vi "real-time recording.vi"() -> ()   [LabVIEW 2012]
doc: "This VI will initialize the FPGA VI and read a user-defined number of samples from a DMA FIFO. When the data acquisition is complete this VI will read status information from the FPGA VI.\n\nFollow these instructions to run the VI.\n\n1. Select your RIO device from the dropdown.\n2. Set the sample period, number of samples to acquire per channel, and DMA block read size. \n\nNote: the block read size should be set to balance load on the host processor and the update rate of the user interface. A small block read size will update the user interface more often but will result in a higher load on the host processor."
uses:
  <vilib>/userdefined/High Color/nirio_resource_hc.ctl
  <vilib>/Analysis/3filter.llb/Butterworth Filter (DBL).vi
  <vilib>/FPGAPlugInAG/sbRIO-9612/niLvFpga_Open_sbRIO-9612.vi
  <vilib>/rvi/interface/common/dynamic/niFpgaDynamicAddResources.vi
  <vilib>/Utility/error.llb/Error Cluster From Error Code.vi
  <vilib>/FPGAPlugInAG/Dynamic/niLvFpga_Run_Dynamic.vi
  <vilib>/rvi/errors/niLvFpgaAdjustHostInterfaceError.vi
  <vilib>/RVI Host/nirviSupport.llb/nirviErrorClusterFromErrorCode.vi
  <vilib>/FPGAPlugInAG/Dynamic/niLvFpga_Close_Dynamic.vi
  <vilib>/rvi/interface/nirviOpenFPGA/nirviOpenFPGA.xnode
  FPGA Bitfiles/bbauvFPGA_FPGATarget2_NI9223User-Contr_AXBjtBmtN8Y.lvbitx
  NI 9223 User-Controlled IO Sampling (FPGA).vi
  <vilib>/rvi/interface/nirviMethod/nirviMethod.xnode
  <vilib>/rvi/interface/nirviReadWriteControl/nirviReadWriteControl.xnode
  <vilib>/rvi/interface/nirviCloseFPGA/nirviCloseFPGA.xnode
  <vilib>/rvi/errors/niLvFpgaMergeErrorWithErrorCode.vi
  <vilib>/rvi/interface/Simulation/niFpgaSimulationCallBeginRW.vi
  <vilib>/FPGAPlugInAG/Dynamic/niLvFpga_ReadFifo_Dynamic.vi
  <vilib>/rvi/interface/nirviMethod/StockFPGA_InlinedMethodWaitForSingleIRQ.vi
  <vilib>/FPGAPlugInAG/Dynamic/niLvFpga_WaitOnIrq_Dynamic.vi
  <vilib>/FPGAPlugInAG/Dynamic/niLvFpga_AcknowledgeIrq_Dynamic.vi
  NiFpgaLv.dll
  <vilib>/FPGAPlugInAG/Dynamic/niLvFpga_ConfigureFifo_Dynamic.vi
  <vilib>/FPGAPlugInAG/Dynamic/niLvFpga_StartFifo_Dynamic.vi
  <vilib>/Analysis/NI_AALBase.lvlib
  <vilib>/Analysis/NI_AALPro.lvlib
panel:
  in  "fake dt2":dbl
  in  "Record?":bool
  in  "Filename":path=path "D/Recorded/US Test/Record 1/test 1.tdms"
  in  "threshold ratio":dbl=3.0
  out "Sidemove":dbl
  out "Forward":dbl
  out "Threshold 3":dbl
  out "Threshold 2":dbl
  out "Threshold 1":dbl
  out "noise index":dbl[](array[numeric])
  out "Threshold 0":dbl
  out "Amplitude Spectrum":waveform(dbl)(graph)
  out "bad signal?":bool
  in  "Min Starting Index":i32=7000
  in  "Portion Duration":i32=1000
  out "amplitude 3":dbl
  out "amplitude 2":dbl
  out "amplitude 1":dbl
  out "amplitude 0":dbl
  in  "noise min":dbl=0.001
  out "Index 3":dbl
  out "Index 2":dbl
  out "Index 1":dbl
  out "Index 0":dbl
  out "current time":timestamp
  in  "Debug":bool=TRUE
  in  "Send to ROS":bool
  out "ROS  Error":bool
  out "dt1":dbl
  out "dt2":dbl
  out "dt3":dbl
  out "pitch":dbl
  out "yaw":dbl
  out "z":dbl
  out "y":dbl
  out "x":dbl
  in  "Mode":T1(ring)=enum."Use Far Field"
  in  "Altitude":dbl=2.0
  in  "Display Filtered Signal":bool=TRUE
  out "Ratio at Index (%)":dbl
  out "Selected Index":i32
  in  "Threshold":dbl=0.1
  in  "low cutoff freq: fl":dbl=20000.0
  in  "high cutoff freq: fh":dbl=30000.0
  out "Yaw Chart":dbl(graph)
  out "Ch0 Signal":dbl[](graph)
  out "#Elements Acquired":u32(graph)
  out "Extracted signal":dbl[][](graph)
  in  "Sampling Duration (us)":u32=2005000
  in  "RIO Device":T2="rio://192.168.0.150/RIO0"
  out "Timed Out":bool
  out "Sample Gated":bool
  out "Overwrite":bool
  in  "Acquisition Stop":bool
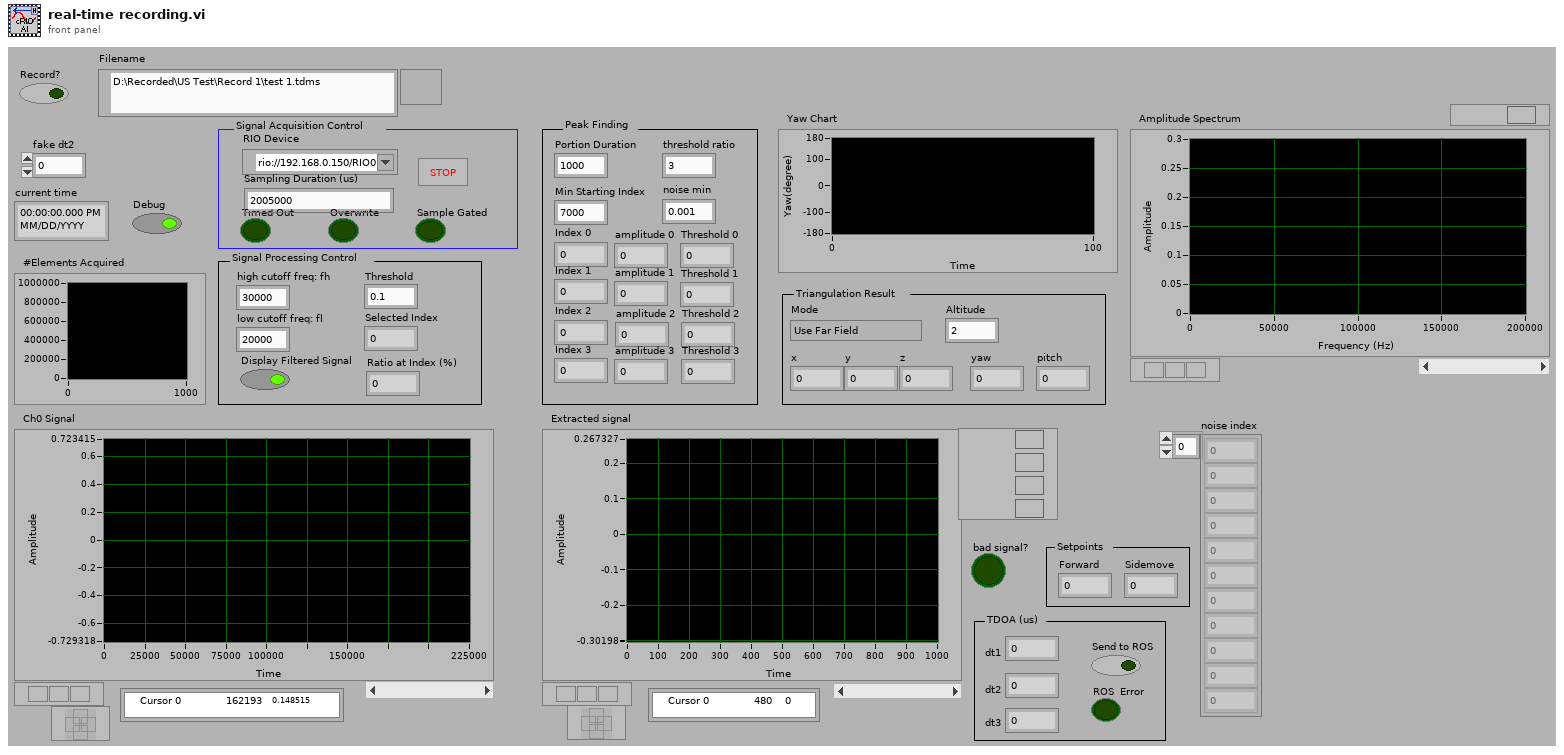
[diagram p1: front panel]
types:
  T1 = enum16{"Use Near Field", "Use Far Field", "Far Field with 3 hydrophones"}
  T2 = typedef "nirio_resource_hc.ctl" = tag
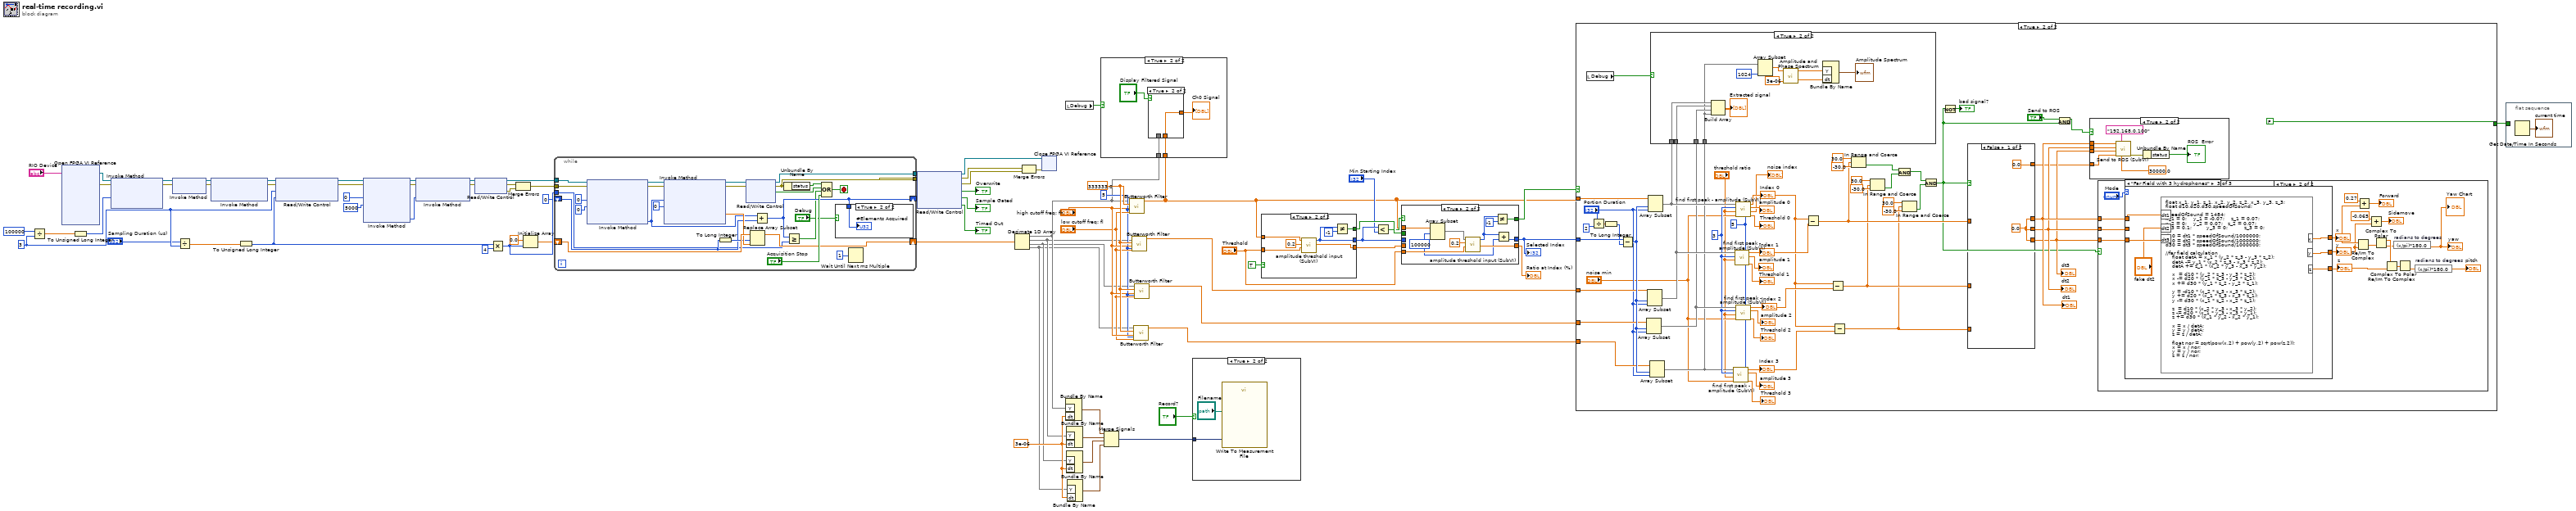
[diagram p0: block diagram]
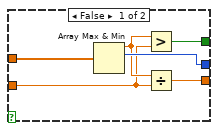
[diagram p6: hidden frame]
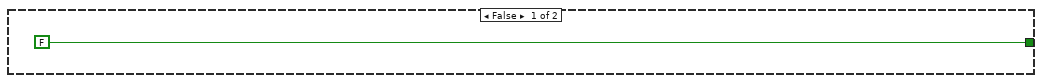
[diagram p7: hidden frame]
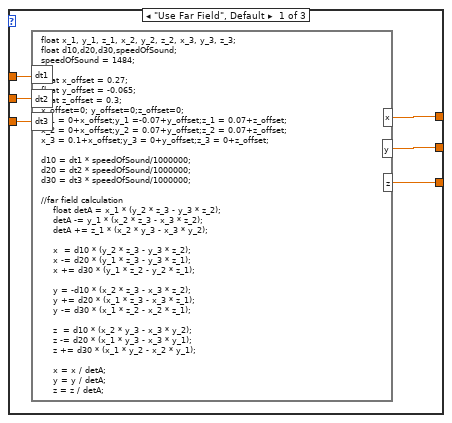
[diagram p9: hidden frame]
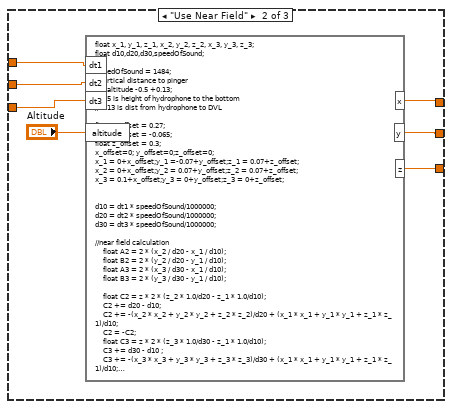
[diagram p10: hidden frame]
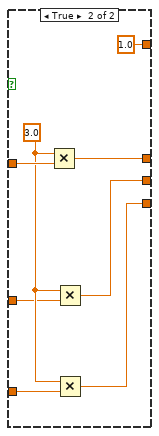
[diagram p12: hidden frame]
diagram:
  w8 = 3e-06
  w16 = 5
  w22 = 333333.0
  w36 = u32 3
  n1 = Divide(x=u32 100000, y=w36) -> (x/y=w69:dbl)
  n2 = xnode "Open FPGA VI Reference"("resource name"="RIO Device") -> ("FPGA VI Reference Out"=w72:refnum<k20>, "error out"=w71:errorcluster)  [unwired: 1 in]
  n3 = To Unsigned Long Integer(number=w69) -> (unsigned 32bit integer=w70:u32)
  n4 = xnode "Invoke Method"("FPGA VI Reference In"=w72, "error in"=w71, "Requested Depth"=w70) -> ("FPGA VI Reference Out"=w74:refnum<k20>, "error out"=w73:errorcluster)  [unwired: 1 out]
  n5 = xnode "Invoke Method"("FPGA VI Reference In"=w74, "error in"=w73) -> ("FPGA VI Reference Out"=w63:refnum<k20>, "error out"=w62:errorcluster)
  n6 = Divide(x="Sampling Duration (us)", y=w36) -> (x/y=w34:dbl)
  n7 = xnode "Invoke Method"("FPGA VI Reference In"=w63, "error in"=w62) -> ("FPGA VI Reference Out"=w39:refnum<k20>, "error out"=w38:errorcluster)  [unwired: 1 in]
  n8 = To Unsigned Long Integer(number=w34) -> (unsigned 32bit integer=w32:u32)
  n9 = xnode "Read/Write Control"("FPGA VI Reference In"=w39, "error in"=w38, "Sample Period (uSec)"=w36, "Number of Samples"=w32) -> ("FPGA VI Reference Out"=w53:refnum<k20>, "error out"=w52:errorcluster)
  n10 = xnode "Invoke Method"("FPGA VI Reference In"=w53, "error in"=w52, "IRQ Number(s)"=0, "Timeout (ms)"=5000) -> ("FPGA VI Reference Out"=w50:refnum<k20>, "error out"=w51:errorcluster, "IRQ(s) Asserted"=w47:i32)  [unwired: 1 out]
  n11 = xnode "Invoke Method"("FPGA VI Reference In"=w50, "error in"=w51, "IRQ Number(s)"=w47) -> ("FPGA VI Reference Out"=w49:refnum<k20>, "error out"=w48:errorcluster)
  n12 = xnode "Read/Write Control"("FPGA VI Reference In"=w49, "error in"=w48) -> ("FPGA VI Reference Out"=w41:refnum<k20>, "error out"=w55:errorcluster, "Error Out"=w54:errorcluster)
  n13 = Multiply(x=w32, y=u32 4) -> (x*y=w66:u32)
  n14 = Merge Errors(w55, w54) -> (w40:errorcluster)
  n15 = Initialize Array(sgl 0.0, w66) -> (w42:sgl[])
  n16 = while {
    tunnel: w41 -> [w88]
    tunnel: w40 -> [w87]
    tunnel: [w96] -> w61
    tunnel: [w95] -> w60
    shift-right: [w78] -> _
    shift-left: u32 0 -> [w89]
    tunnel: w66 -> [w81]
    shift-right: [w91] -> w33
    shift-left: w42 -> [w97]
    stop <- w98 stop-if-true
    n17 = xnode "Invoke Method"("FPGA VI Reference In"=w88, "error in"=w87, "Number of Elements"=u32 0, "Timeout (ms)"=0) -> ("FPGA VI Reference Out"=w86:refnum<k20>, "error out"=w85:errorcluster, "Elements Remaining"=w79:u32)  [unwired: 1 out]
    n18 = xnode "Invoke Method"("FPGA VI Reference In"=w86, "error in"=w85, "Number of Elements"=w79, "Timeout (ms)"=0) -> ("FPGA VI Reference Out"=w101:refnum<k20>, "error out"=w100:errorcluster, "Data"=w92:sgl[])  [unwired: 1 out]
    n19 = To Long Integer(number=w89) -> (32bit integer=w90:i32)
    n20 = xnode "Read/Write Control"("FPGA VI Reference In"=w101, "error in"=w100) -> ("FPGA VI Reference Out"=w96:refnum<k20>, "error out"=w95:errorcluster, "Error"=w80:bool)  [unwired: 1 out]
    n21 = Replace Array Subset(array=w97, new element=w92, index=w90) -> (w91:sgl[])
    n22 = Add(x=w79, y=w89) -> (x+y=w78:u32)
    n23 = Unbundle By Name(w95) -> ("status"=w82:bool)
    n24 = Greater Or Equal?(x=w78, y=w81) -> (x >= y?=w77:bool)
    n25 = Compound Arithmetic op=OR(w82, w80, w77, "Acquisition Stop") -> (w98:bool)
    n26 = case shown="True" "Debug" {
      tunnel: w78 -> [_ w102]
      frame False {
      }
      frame True {
        "#Elements Acquired" <- w102
      }
    }
    n27 = Wait Until Next ms Multiple(millisecond multiple=u32 1) -> ()  [unwired: 1 out]
  }
  n28 = xnode "Read/Write Control"("FPGA VI Reference In"=w61, "error in"=w60) -> ("FPGA VI Reference Out"=w65:refnum<k20>, "error out"=w56:errorcluster, "Error Out"=w57:errorcluster, "Overwrite"=→"Overwrite":bool, "Sample Gated"=→"Sample Gated":bool, "Timed Out"=→"Timed Out":bool)
  n29 = Decimate 1D Array(w33) -> (w4:sgl[], w3:sgl[], w2:sgl[], w1:sgl[])
  n30 = Merge Errors(w56, w57) -> (w64:errorcluster)
  n31 = xnode "Close FPGA VI Reference"("FPGA VI Reference In"=w65, "error in"=w64) -> ()  [unwired: 1 out]
  n32 = local read "Debug"() -> (w14:bool)
  n33 = Bundle By Name("Y"=w4, "dt"=w8) -> (w11:waveform(sgl))  [unwired: 1 in]
  n34 = Bundle By Name("Y"=w3, "dt"=w8) -> (w10:waveform(sgl))  [unwired: 1 in]
  n35 = Bundle By Name("Y"=w2, "dt"=w8) -> (w9:waveform(sgl))  [unwired: 1 in]
  n36 = Bundle By Name("Y"=w1, "dt"=w8) -> (w7:waveform(sgl))  [unwired: 1 in]
  n37 = Merge Signals(w11, w10, w9, w7) -> (w6:dynamicdata)
  n38 = call-poly <vilib>:"Butterworth Filter.vi"("order"=w16, "low cutoff freq: fl"="low cutoff freq: fl", "high cutoff freq: fh"="high cutoff freq: fh", "sampling freq: fs"=w22, "X"=w4) -> ("Filtered X"=w12:dbl[])  [unwired: 3 in, 1 out]
  n39 = case shown="True" w14 {
    tunnel: w12 -> [_ w104]
    tunnel: w4 -> [_ w103]
    frame False {
    }
    frame True {
      n40 = case shown="True" "Display Filtered Signal" {
        tunnel: w103 -> [w107 _]
        tunnel: [w107 w108] -> w105
        tunnel: w104 -> [_ w108]
        frame False {
        }
        frame True {
        }
      }
      "Ch0 Signal" <- w105
    }
  }
  n41 = call-poly <vilib>:"Butterworth Filter.vi"("order"=w16, "low cutoff freq: fl"="low cutoff freq: fl", "high cutoff freq: fh"="high cutoff freq: fh", "sampling freq: fs"=w22, "X"=w3) -> ("Filtered X"=w19:dbl[])  [unwired: 3 in, 1 out]
  n42 = call-poly <vilib>:"Butterworth Filter.vi"("order"=w16, "low cutoff freq: fl"="low cutoff freq: fl", "high cutoff freq: fh"="high cutoff freq: fh", "sampling freq: fs"=w22, "X"=w1) -> ("Filtered X"=w17:dbl[])  [unwired: 3 in, 1 out]
  n43 = call-poly <vilib>:"Butterworth Filter.vi"("order"=w16, "low cutoff freq: fl"="low cutoff freq: fl", "high cutoff freq: fh"="high cutoff freq: fh", "sampling freq: fs"=w22, "X"=w2) -> ("Filtered X"=w18:dbl[])  [unwired: 3 in, 1 out]
  n44 = case shown="True" "Record?" {
    tunnel: w6 -> [_ w110]
    frame False {
    }
    frame True {
      n45 = call "Write To Measurement File"("Signals"=w110, "Filename"="Filename") -> ()  [unwired: 15 in, 3 out]
    }
  }
  n46 = case shown="True" TRUE {
    tunnel: w12 -> [w116 w123]
    tunnel: [w113 w120] -> w28
    tunnel: [w114 w119] -> w25
    tunnel: [w115 w118] -> w30
    tunnel: "Threshold" -> [w111 w117]
    frame False {
      n47 = Array Max & Min(array=w116) -> (max value=w112:dbl, max index (indices)=w114:i32)  [unwired: 2 out]
      n48 = Greater?(x=w112, y=w111) -> (0:w115:bool)
      n49 = Divide(x=w112, y=w111) -> (x/y=w113:dbl)
    }
    frame True {
      n50 = call "amplitude threshold input (SubVI).vi"("threshold"=w117, "%max amplitude"=0.2, "Array"=w123) -> ("actual ratio (%)"=w120:dbl, "Index"=w119:i32)  [unwired: 7 in]
      n51 = Not Equal?(x=w119, y=-1) -> (x != y?=w118:bool)
    }
  }
  n52 = Less?(x=w25, y="Min Starting Index") -> (x < y?=w29:bool)
  n53 = case shown="True" w29 {
    tunnel: w30 -> [w126 _]
    tunnel: w28 -> [w124 _]
    tunnel: w12 -> [_ w136]
    tunnel: "Threshold" -> [_ w132]
    tunnel: [w126 w131] -> w23
    tunnel: [w125 w129] -> w24
    tunnel: [w124 w130] -> w26
    tunnel: w25 -> [w125 _]
    frame False {
    }
    frame True {
      w127 = 100000
      n54 = Array Subset(array=w136, index=w127) -> (w133:dbl[])  [unwired: 1 in]
      n55 = call "amplitude threshold input (SubVI).vi"("threshold"=w132, "%max amplitude"=0.2, "Array"=w133) -> ("actual ratio (%)"=w130:dbl, "Index"=w128:i32)  [unwired: 7 in]
      n56 = Not Equal?(x=w128, y=-1) -> (x != y?=w131:bool)
      n57 = Add(x=w128, y=w127) -> (x+y=w129:i32)
    }
  }
  "Ratio at Index (%)" <- w26
  "Selected Index" <- w24
  n58 = case shown="True" w23 {
    tunnel: w19 -> [_ w190]
    tunnel: w18 -> [_ w189]
    tunnel: w17 -> [_ w188]
    tunnel: w12 -> [_ w187]
    tunnel: w24 -> [_ w186]
    tunnel: [FALSE FALSE] -> w13
    frame False {
    }
    frame True {
      w138 = 5
      w151 = 3
      n59 = local read "Debug"() -> (w181:bool)
      n60 = Divide(x="Portion Duration", y=2) -> (x/y=w183:dbl)
      n61 = To Long Integer(number=w183) -> (32bit integer=w182:i32)
      n62 = Subtract(x=w186, y=w182) -> (x-y=w191:i32)
      n63 = Array Subset(array=w189, index=w191, length="Portion Duration") -> (w152:dbl[])
      n64 = Array Subset(array=w190, index=w191, length="Portion Duration") -> (w156:dbl[])
      n65 = Array Subset(array=w187, index=w191, length="Portion Duration") -> (w158:dbl[])
      n66 = Array Subset(array=w188, index=w191, length="Portion Duration") -> (w150:dbl[])
      n67 = case shown="True" w181 {
        tunnel: w156 -> [_ w257]
        tunnel: w152 -> [_ w256]
        tunnel: w150 -> [_ w247]
        tunnel: w158 -> [_ w255]
        frame False {
        }
        frame True {
          n68 = Build Array(w255, w257, w256, w247) -> (→"Extracted signal":dbl[][])
          n69 = Array Subset(array=w247, length=1024) -> (w251:dbl[])  [unwired: 1 in]
          n70 = call <vilib>:"Amplitude and Phase Spectrum.vi"("dt"=3e-06, "Signal (V)"=w251) -> ("df"=w248:dbl, "Amp Spectrum Mag (Vrms)"=w249:dbl[])  [unwired: 1 in, 1 out]
          n71 = Bundle By Name("Y"=w249, "dt"=w248) -> (→"Amplitude Spectrum":waveform(dbl))  [unwired: 1 in]
        }
      }
      n72 = call "find first peak - amplitude (SubVI).vi"("Noise length"=w138, "Noise min"="noise min", "threshold ratio"="threshold ratio", "width"=w151, "Array"=w150) -> ("Peak threshold"=→"Threshold 3":dbl, "peak amplitude"=→"amplitude 3":dbl, "Index"=w149:dbl)  [unwired: 2 in, 2 out]
      "Index 3" <- w149
      n73 = call "find first peak - amplitude (SubVI).vi"("Noise length"=w138, "threshold ratio"="threshold ratio", "width"=w151, "Array"=w156) -> ("Peak threshold"=→"Threshold 1":dbl, "peak amplitude"=→"amplitude 1":dbl, "Index"=w155:dbl)  [unwired: 3 in, 2 out]
      "Index 1" <- w155
      n74 = call "find first peak - amplitude (SubVI).vi"("Noise length"=w138, "Noise min"="noise min", "threshold ratio"="threshold ratio", "width"=w151, "Array"=w158) -> ("Peak threshold"=→"Threshold 0":dbl, "noise index"=→"noise index":dbl[], "peak amplitude"=→"amplitude 0":dbl, "Index"=w145:dbl)  [unwired: 2 in, 1 out]
      "Index 0" <- w145
      n75 = call "find first peak - amplitude (SubVI).vi"("Noise length"=w138, "Noise min"="noise min", "threshold ratio"="threshold ratio", "width"=w151, "Array"=w152) -> ("Peak threshold"=→"Threshold 2":dbl, "peak amplitude"=→"amplitude 2":dbl, "Index"=w153:dbl)  [unwired: 2 in, 2 out]
      "Index 2" <- w153
      n76 = Subtract(x=w145, y=w155) -> (x-y=w177:dbl)
      n77 = Subtract(x=w145, y=w153) -> (x-y=w174:dbl)
      n78 = Subtract(x=w145, y=w149) -> (x-y=w171:dbl)
      n79 = In Range and Coerce(upper limit=30.0, x=w177, lower limit=-30.0) -> (In Range?=w170:bool)  [unwired: 1 out]
      n80 = In Range and Coerce(upper limit=30.0, x=w174, lower limit=-30.0) -> (In Range?=w169:bool)  [unwired: 1 out]
      n81 = And(x=w170, y=w169) -> (x .and. y?=w168:bool)
      n82 = In Range and Coerce(upper limit=30.0, x=w171, lower limit=-30.0) -> (In Range?=w167:bool)  [unwired: 1 out]
      n83 = And(x=w168, y=w167) -> (x .and. y?=w159:bool)
      n84 = Not(x=w159) -> (.not. x?=→"bad signal?":bool)
      n85 = case shown="False" w159 {
        tunnel: w177 -> [_ w246]
        tunnel: w174 -> [_ w244]
        tunnel: w171 -> [_ w243]
        tunnel: [w237 w242] -> w164
        tunnel: [w237 w241] -> w163
        tunnel: [w237 w240] -> w162
        tunnel: [0.0 1.0] -> w161
        frame False {
          w237 = 0.0
        }
        frame True {
          w245 = 3.0
          n86 = Multiply(x=w245, y=w246) -> (x*y=w242:dbl)
          n87 = Multiply(x=w245, y=w244) -> (x*y=w241:dbl)
          n88 = Multiply(x=w245, y=w243) -> (x*y=w240:dbl)
        }
      }
      "dt1" <- w164
      "dt2" <- w163
      "dt3" <- w162
      n89 = And(x="Send to ROS", y=w159) -> (x .and. y?=w160:bool)
      n90 = case shown="True" w160 {
        tunnel: w164 -> [_ w232]
        tunnel: w163 -> [_ w231]
        tunnel: w162 -> [_ w230]
        tunnel: w161 -> [_ w229]
        frame False {
        }
        frame True {
          n91 = call "Send to ROS (SubVI).vi"("frequency"=30000.0, "ROS IP"="192.168.0.100", "Good signal?"=w229, "dt 3"=w230, "dt2"=w231, "dt 1"=w232) -> ("error out"=w235:errorcluster)  [unwired: 5 in]
          n92 = Unbundle By Name(w235) -> ("status"=→"ROS  Error":bool)
        }
      }
      n93 = case shown="True" w159 {
        tunnel: w164 -> [_ w200]
        tunnel: w163 -> [_ w199]
        tunnel: w162 -> [_ w198]
        frame False {
        }
        frame True {
          n94 = case shown="\"Far Field with 3 hydrophones\"" "Mode" {
            tunnel: [w215 w222 w228] -> w197
            tunnel: [w214 w221 w227] -> w194
            tunnel: [w213 w220 w226] -> w204
            tunnel: w200 -> [w212 w218 w225]
            tunnel: w199 -> [w211 w217 _]
            tunnel: w198 -> [w210 w216 w224]
            frame "Use Far Field", Default {
              n95 = formula code="float x_1, y_1, z_1, x_2, y_2, z_2, x_3, y_3, z_3;\nfloat d10,d20,d30,speedOfSound;\nspeedOfSound = 1484;\n\nfloat x_offset = 0.27;\nfloat y_offset = -0.065;\nfloat z_offset = 0.3;\nx_offset=0; y_offset=0;z_offset=0;\nx_1 = 0+x_offset;y_1 =-0.07+y_offset;z_1 = 0.07+z_offset;\nx_2 = 0+x_offset;y_2 = 0.07+y_offset;z_2 = 0.07+z_offset;\nx_3 = 0.1+x_offset;y_3 = 0+y_offset;z_3 = 0+z_offset;\n\nd10 = dt1 * speedOfSound/1000000;\nd20 = dt2 * speedOfSound/1000000;\nd30 = dt3 * speedOfSound/1000000;\n\n//far field calculation\n    float detA = x_1 * (y_2 * z_3 - y_3 * z_2);\n    detA -= y_1 * (x_2 * z_3 - x_3 * z_2);\n    detA += z_1 * (x_2 * y_3 - x_3 * y_2);\n\n    x  = d10 * (y_2 * z_3 - y_3 * z_2);\n    x -= d20 * (y_1 * z_3 - y_3 * z_1);\n    x += d30 * (y_1 * z_2 - y_2 * z_1);\n\n    y = -d10 * (x_2 * z_3 - x_3 * z_2);\n    y += d20 * (x_1 * z_3 - x_3 * z_1);\n    y -= d30 * (x_1 * z_2 - x_2 * z_1);\n\n    z  = d10 * (x_2 * y_3 - x_3 * y_2);\n    z -= d20 * (x_1 * y_3 - x_3 * y_1);\n    z += d30 * (x_1 * y_2 - x_2 * y_1);\n\n    x = x / detA;\n    y = y / detA;\n    z = z / detA;\n\n    float nor = sqrt(pow(x,2) + pow(y,2) + pow(z,2));\n    x = x / nor;\n    y = y / nor;\n    z = z / nor;"("dt1"=w212, "dt2"=w211, "dt3"=w210) -> ("x"=w215:dbl, "y"=w214:dbl, "z"=w213:dbl)
            }
            frame "Use Near Field" {
              n96 = formula code="float x_1, y_1, z_1, x_2, y_2, z_2, x_3, y_3, z_3;\nfloat d10,d20,d30,speedOfSound;\n\nspeedOfSound = 1484;\n//vertical distance to pinger\nz= altitude -0.5 +0.13;\n// 0.5 is height of hydrophone to the bottom\n// 0.13 is dist from hydrophone to DVL\n\nfloat x_offset = 0.27;\nfloat y_offset = -0.065;\nfloat z_offset = 0.3;\nx_offset=0; y_offset=0;z_offset=0;\nx_1 = 0+x_offset;y_1 =-0.07+y_offset;z_1 = 0.07+z_offset;\nx_2 = 0+x_offset;y_2 = 0.07+y_offset;z_2 = 0.07+z_offset;\nx_3 = 0.1+x_offset;y_3 = 0+y_offset;z_3 = 0+z_offset;\n\n\nd10 = dt1 * speedOfSound/1000000;\nd20 = dt2 * speedOfSound/1000000;\nd30 = dt3 * speedOfSound/1000000;\n\n//near field calculation\n    float A2 = 2 * (x_2 / d20 - x_1 / d10);\n    float B2 = 2 * (y_2 / d20 - y_1 / d10);\n    float A3 = 2 * (x_3 / d30 - x_1 / d10);\n    float B3 = 2 * (y_3 / d30 - y_1 / d10);\n    \n    float C2 = z * 2 * (z_2 * 1.0/d20 - z_1 * 1.0/d10);\n    C2 += d20 - d10;\n    C2 += -(x_2 * x_2 + y_2 * y_2 + z_2 * z_2)/d20 + (x_1 * x_1 + y_1 * y_1 + z_1 * z_1)/d10;\n    C2 = -C2;\n    float C3 = z * 2 * (z_3 * 1.0/d30 - z_1 * 1.0/d10);\n    C3 += d30 - d10 ;\n    C3 += -(x_3 * x_3 + y_3 * y_3 + z_3 * z_3)/d30 + (x_1 * x_1 + y_1 * y_1 + z_1 * z_1)/d10;\n    C3 = -C3;\n\n    if (A2*B3 == A3*B2) {\n        x = 0;\n        y = 0;\n    }\n    else {\n        x = (C2 * B3 - C3 * B2) / (A2 * B3 - A3 * B2);\n        y = (C3 * A2 - C2 * A3) / (B3 * A2 - B2 * A3);\n    }"("dt1"=w218, "dt2"=w217, "dt3"=w216, "altitude"="Altitude") -> ("x"=w222:dbl, "y"=w221:dbl, "z"=w220:dbl)
            }
            frame "Far Field with 3 hydrophones" {
              n97 = formula code="float x_1, y_1, z_1, x_2, y_2, z_2, x_3, y_3, z_3;\nfloat d10,d20,d30,speedOfSound;\n\nspeedOfSound = 1484;\nx_1 = 0;    y_1 = -0.07;    z_1 = 0.07;\nx_2 = 0;    y_2 = 0.07;   z_2 = 0.07;\nx_3 = 0.1;         y_3 = 0;          z_3 = 0;\n\nd10 = dt1 * speedOfSound/1000000;\nd20 = dt2 * speedOfSound/1000000;\nd30 = dt3 * speedOfSound/1000000;\n\n//far field calculation\n    float detA = x_1 * (y_2 * z_3 - y_3 * z_2);\n    detA -= y_1 * (x_2 * z_3 - x_3 * z_2);\n    detA += z_1 * (x_2 * y_3 - x_3 * y_2);\n\n    x  = d10 * (y_2 * z_3 - y_3 * z_2);\n    x -= d20 * (y_1 * z_3 - y_3 * z_1);\n    x += d30 * (y_1 * z_2 - y_2 * z_1);\n\n    y = -d10 * (x_2 * z_3 - x_3 * z_2);\n    y += d20 * (x_1 * z_3 - x_3 * z_1);\n    y -= d30 * (x_1 * z_2 - x_2 * z_1);\n\n    z  = d10 * (x_2 * y_3 - x_3 * y_2);\n    z -= d20 * (x_1 * y_3 - x_3 * y_1);\n    z += d30 * (x_1 * y_2 - x_2 * y_1);\n\n    x = x / detA;\n    y = y / detA;\n    z = z / detA;\n\n    float nor = sqrt(pow(x,2) + pow(y,2) + pow(z,2));\n    x = x / nor;\n    y = y / nor;\n    z = z / nor;"("dt1"=w225, "dt2"="fake dt2", "dt3"=w224) -> ("x"=w228:dbl, "y"=w227:dbl, "z"=w226:dbl)
            }
          }
          "x" <- w197
          "y" <- w194
          "z" <- w204
          n98 = Re/Im To Complex(1:w194, 2:w197) -> (0:w202:cdb)
          n99 = Add(x=0.27, y=w197) -> (x+y=→"Forward":dbl)
          n100 = Add(x=-0.065, y=w194) -> (x+y=→"Sidemove":dbl)
          n101 = Complex To Polar(r * e^(i*theta)=w202) -> (r=w205:dbl, theta=w203:dbl)
          n102 = Re/Im To Complex(1:w204, 2:w205) -> (0:w206:cdb)
          n103 = expression code="(x/pi)*180.0"(w203) -> (→"yaw" →"Yaw Chart":dbl)
          n104 = Complex To Polar(r * e^(i*theta)=w206) -> (theta=w208:dbl)  [unwired: 1 out]
          n105 = expression code="(x/pi)*180.0"(w208) -> (→"pitch":dbl)
        }
      }
    }
  }
  n106 = flat-sequence {
    tunnel: w13 -> [_]
    frame #0 {
      n107 = Get Date/Time In Seconds() -> (seconds since 1Jan1904=→"current time":timestamp)
    }
  }
